vi "Hardware - NI 9758-2 (PFI-LS) Host.vi"() -> ()   [LabVIEW 2015, in "ECS-Host.lvlib"]
uses:
  ECS-Host.lvlib
panel:
  in  "_Tab Control":T1(tab)
  in  "DisableOnCrit":bool caption="Disable On Crit?"
  in  "PFIMaxDuration":sgl caption="[DBTDC]"
  in  "PFIMinDuration":sgl caption="[DBTDC]"
  in  "PFIWindowEnd":sgl caption="[DBTDC]"
  in  "PFIWindowStart":sgl caption="[DBTDC]"
  in  "PFI1RecircAlways":bool
  in  "PFI1Enable":bool
  in  "PFI2RecircAlways":bool
  in  "PFI2Enable":bool
  in  "PFI3RecircAlways":bool
  in  "PFI3Enable":bool
  in  "PFI4RecircAlways":bool
  in  "PFI4Enable":bool
  in  "PFI1Phase1FirstPeakEnable":bool
  in  "PFI2Phase1FirstPeakEnable":bool
  in  "PFI3Phase1FirstPeakEnable":bool
  in  "PFI4Phase1FirstPeakEnable":bool
  out "_PFI_IPhaseIndex":string[](array[string])
  in  "IPhaseCurrent":sgl[](array[numeric]) format="%#.3f"
  in  "IPhaseDuration":sgl[](array[numeric]) format="%#.3f"
  out "ModulePresent":bool
  in  "ModuleEnable":bool
  out "ModuleRev":string
  in  "OneShot":bool
  in  "OneShotSelect":enum32{"a", "b", "c", "d", "e"}(ring)
  in  "OneShotDuration":sgl caption="msec" format="%#.3f"
  out "LS4Enabled":bool caption="Enable"
  out "LS3Enabled":bool caption="Enable"
  out "LS2Enabled":bool caption="Enable"
  out "LS1Enabled":bool caption="Enable"
  out "LS1DC":sgl caption="[]"
  out "LS4DC":sgl caption="[V]"
  out "LS3DC":sgl caption="[V]"
  out "LS2DC":sgl caption="[V]"
  out "LS4Freq":sgl caption="[]" format="%#.2f"
  out "LS3Freq":sgl caption="[]" format="%#.2f"
  out "LS1Freq":sgl caption="[]" format="%#.2f"
  out "LS2Freq":sgl caption="[]" format="%#.2f"
  out "_LS Assignment":string[](array[string]) caption="Actuators"
  out "_LS Index":string[](array[string]) caption="PFI/LS1 Chan"
  out "FPGAReadError":bool
  out "FPGAWriteError":bool
  in  "OpenFaultOverride":bool
  in  "FaultClear":bool
  out "LS4ShortCircuitFault":bool caption="Enable"
  out "LS3ShortCircuitFault":bool caption="Enable"
  out "LS2ShortCircuitFault":bool caption="Enable"
  out "LS1ShortCircuitFault":bool caption="Enable"
  out "LS4OpenCircuitFault":bool caption="Enable"
  out "LS3OpenCircuitFault":bool caption="Enable"
  out "LS2OpenCircuitFault":bool caption="Enable"
  out "LS1OpenCircuitFault":bool caption="Enable"
  out "PFI4ShortCircuitFault":bool caption="Enable"
  out "PFI3ShortCircuitFault":bool caption="Enable"
  out "PFI2ShortCircuitFault":bool caption="Enable"
  out "PFI1ShortCircuitFault":bool caption="Enable"
  out "PFI4OpenCircuitFault":bool caption="Enable"
  out "PFI3OpenCircuitFault":bool caption="Enable"
  out "PFI2OpenCircuitFault":bool caption="Enable"
  out "PFI1OpenCircuitFault":bool caption="Enable"
  # "PFI Channel 1"
  # "PFI Channel 2"
  # "PFI Channel 3"
  # "PFI Channel 4"
  # "PFI Mod 1"
  # "Current Set"
  # "[Amps]"
  # "Duration"
  # "[msec]"
  # "Status"
  # "DC [%]"
  # "Freq [Hz]"
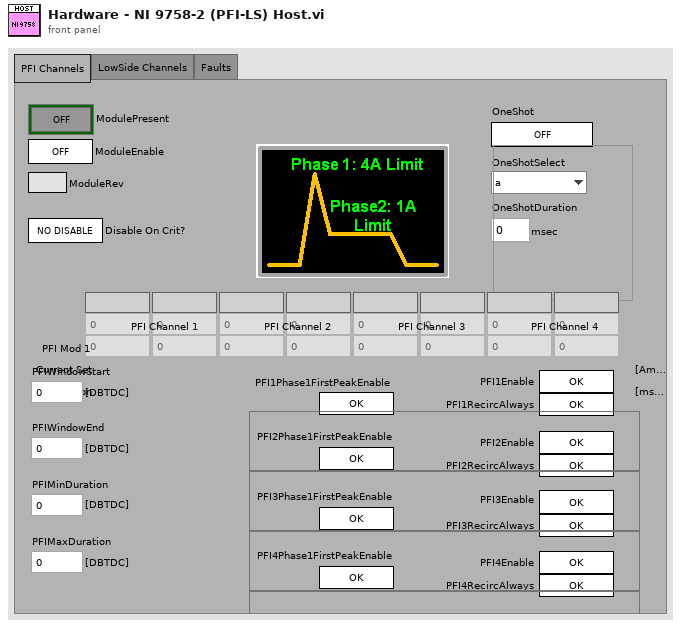
[diagram p1: front panel]
types:
  T1 = enum32{"PFI Channels", "LowSide Channels", "Faults"}
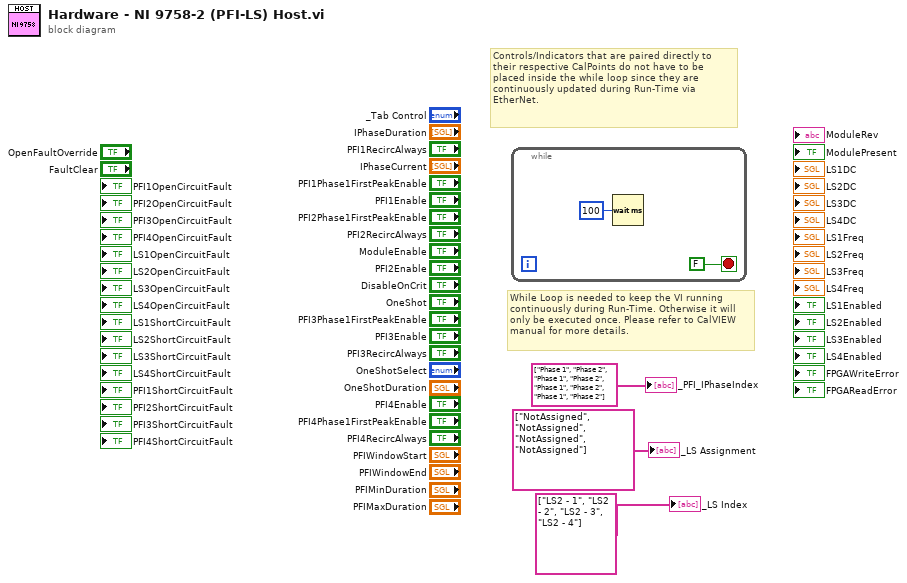
[diagram p0: block diagram]
diagram:
  # "While Loop is needed to keep the VI running\ncontinuously during Run-Time. Otherwise it will only be executed once. Please refer to CalVIEW manual for more details."
  # "Controls/Indicators that are paired directly to their respective CalPoints do not have to be placed inside the while loop since they are continuously updated during Run-Time via EtherNet."
  n1 = while {
    stop <- FALSE stop-if-true
    n2 = Wait (ms)(milliseconds to wait=u32 100) -> ()  [unwired: 1 out]
  }
  "_PFI_IPhaseIndex" <- string[] ["Phase 1", "Phase 2", "Phase 1", "Phase 2", "Phase 1", "Phase 2", "Phase 1", "Phase 2"] ("_PFIIPhaseIndex 2")
  "_LS Index" <- string[] ["LS2 - 1", "LS2 - 2", "LS2 - 3", "LS2 - 4"] ("Array")
  "_LS Assignment" <- string[] ["NotAssigned", "NotAssigned", "NotAssigned", "NotAssigned"] ("Array")
